vi "Derivative (single).vi"(8 "error in (no error)":errorcluster, 9 "Type":enum16{"dy/dx vs x", "dx/dy vs y"}(ring), 11 "XY-data":cluster{"X-array":dbl[], "Y-array":dbl[]}) -> (0 "error out":errorcluster, 2 "Differential out":cluster{"X-array":dbl[], "Y-array":dbl[]} {"Y-array" format="%.2p"; "X-array" format="%.2p"}, 3 "XY-data out":cluster{"X-array":dbl[], "Y-array":dbl[]})   [LabVIEW 2019, in "xy_utilities.lvlib"]
doc: "Performs numerical differentiation of <b>XY-data</b> using the finite difference method.\n\n<b>Interval</b> is the range over which the finite difference is calculated.\n<b>Interval Units</b> defines the units of the <b>Interval</b> to be the number of points or the same units as the x (or y) data.\n<b>Type</b> specifies taking a derivative with respect to x or y.\n\nWire data to the data input to determine the polymorphic instance to use or manually select the instance."
uses:
  xy_utilities.lvlib
  <vilib>/Analysis/NI_AALPro.lvlib
  Swap X and Y (single).vi
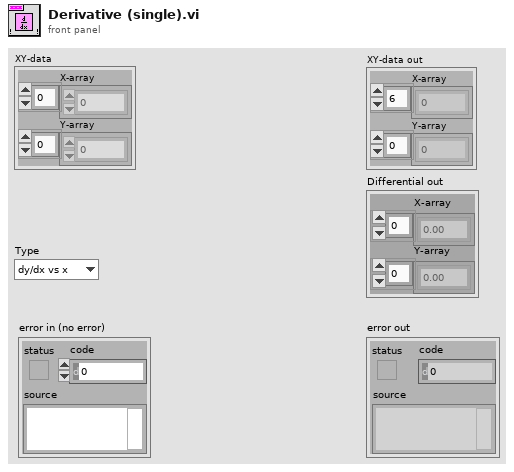
[diagram p1: front panel]
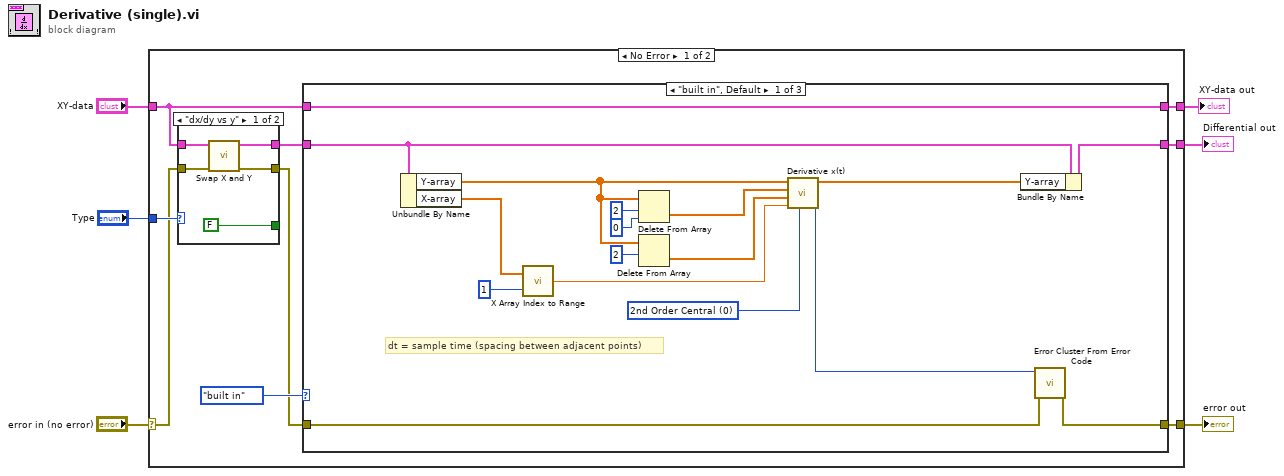
[diagram p0: block diagram]
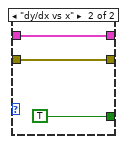
[diagram p2: hidden frame]
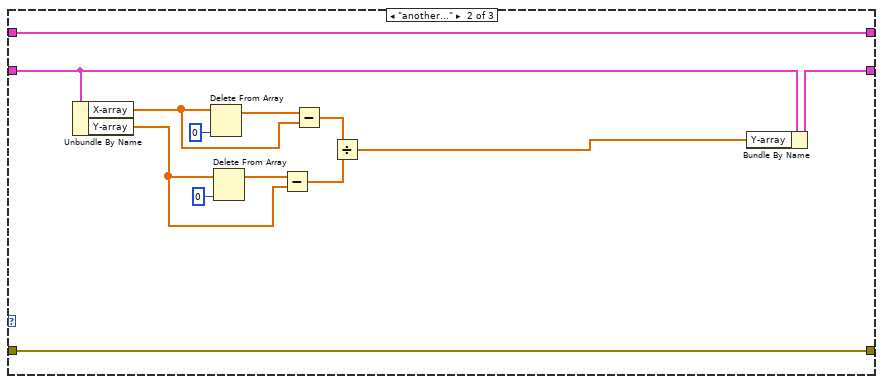
[diagram p3: hidden frame]
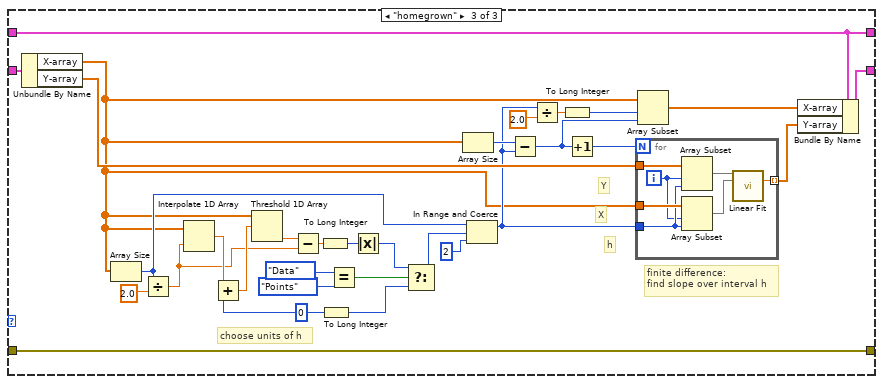
[diagram p4: hidden frame]
diagram:
  n1 = case shown="No Error" "error in (no error)" {
    selector: "error in (no error)" -> [w14 w93]
    tunnel: [w9 w93] -> w5
    tunnel: "XY-data" -> [w13 w92]
    tunnel: [w12 _] -> w3
    tunnel: "Type" -> [w15 _]
    tunnel: [w10 w92] -> w1
    frame No Error {
      n2 = case shown="\"dx/dy vs y\"" w15 {
        tunnel: w13 -> [w20 w23]
        tunnel: [w19 w23] -> w11
        tunnel: [w18 w22] -> w7
        tunnel: w14 -> [w17 w22]
        tunnel: [FALSE ("dy/dx vs x") TRUE ("dy/dx vs x")] -> _
        frame "dx/dy vs y" {
          n3 = call-poly "Swap X and Y.vi"("error in (no error)"=w17, "XY-data"=w20) -> ("error out"=w18:errorcluster, "XY-data out"=w19:cluster{"X-array":dbl[], "Y-array":dbl[]})  [unwired: 8 in]
        }
        frame "dy/dx vs x" {
        }
      }
      n4 = case shown="\"built in\", Default" enum16{"built in", "another...", "homegrown"}."built in" ("Subset Method") {
        tunnel: w13 -> [w37 w52 w67]
        tunnel: [w36 w44 w54] -> w12
        tunnel: w11 -> [w38 w46 w55]
        tunnel: [w37 w52 w67] -> w10
        tunnel: [w39 w53 w66] -> w9
        tunnel: w7 -> [w40 w53 w66]
        frame "built in", Default {
          w31 = u16 0 items=["2nd Order Central", "4th Order Central", "Forward", "Backward"] ("method")
          # "dt = sample time (spacing between adjacent points)"
          n5 = Unbundle By Name(w38) -> ("Y-array"=w30:dbl[], "X-array"=w35:dbl[])
          n6 = call "X Array Index to Range.vi"("X Range (points)"=1 ("X Range (index)"), "X-array"=w35) -> ("X Range (data)"=w34:dbl)
          n7 = Delete From Array(array=w30, length=2 ("index"), index=0 ("length")) -> (deleted portion=w33:dbl[])  [unwired: 1 out]
          n8 = Delete From Array(array=w30, length=2 ("index")) -> (deleted portion=w26:dbl[])  [unwired: 1 in, 1 out]
          n9 = call <vilib>:"Derivative x(t).vi"("method"=w31, "dt"=w34, "Final Condition"=w26, "Initial Condition"=w33, "X"=w30) -> ("error"=w32:i32, "dX/dt"=w25:dbl[])  [unwired: 5 in]
          n10 = Bundle By Name(cluster=w38, "Y-array"=w25) -> (w36:cluster{"X-array":dbl[], "Y-array":dbl[]})
          n11 = call <vilib>:"Error Cluster From Error Code.vi"("error in (no error)"=w40, "error code (0)"=w32) -> ("error out"=w39:errorcluster)  [unwired: 7 in]
        }
        frame "another..." {
          n12 = Unbundle By Name(w46) -> ("X-array"=w41:dbl[], "Y-array"=w49:dbl[])
          n13 = Delete From Array(array=w41, index=0) -> (array with subset deleted=w51:dbl[])  [unwired: 1 in, 1 out]
          n14 = Delete From Array(array=w49, index=0) -> (array with subset deleted=w50:dbl[])  [unwired: 1 in, 1 out]
          n15 = Subtract(x=w50, y=w49) -> (x-y=w47:dbl[])
          n16 = Subtract(x=w51, y=w41) -> (x-y=w48:dbl[])
          n17 = Divide(x=w48, y=w47) -> (x/y=w45:dbl[])
          n18 = Bundle By Name(cluster=w46, "Y-array"=w45) -> (w44:cluster{"X-array":dbl[], "Y-array":dbl[]})
        }
        frame "homegrown" {
          w56 = 0 ("number")
          # "choose units of h"
          # "h"
          # "finite difference:\nfind slope over interval h"
          # "Y"
          # "X"
          n19 = Unbundle By Name(w55) -> ("X-array"=w58:dbl[], "Y-array"=w68:dbl[])
          n20 = Array Size(array=w58) -> (size(s)=w65:i32)
          n21 = Divide(x=w65, y=2.0) -> (x/y=w59:dbl)
          n22 = Interpolate 1D Array(1:w59, 2:w58) -> (0:w60:dbl)
          n23 = Add(x=w60, y=w56) -> (x+y=w74:dbl)
          n24 = Threshold 1D Array(2:w74, 3:w58) -> (0:w76:dbl)  [unwired: 1 in]
          n25 = Subtract(x=w76, y=w59) -> (x-y=w75:dbl)
          n26 = To Long Integer(number=w75) -> (32bit integer=w73:i32)
          n27 = To Long Integer(number=w56) -> (32bit integer=w70:i32)
          n28 = Equal?(x=enum16{"Points", "Data"}."Data" ("Interval Units"), y=enum16{"Points", "Data"}."Points") -> (x = y?=w71:bool)
          n29 = Absolute Value(x=w73) -> (abs(x)=w63:i32)
          n30 = Select(t=w63, s=w71, f=w70) -> (s? t:f=w62:i32)
          n31 = Array Size(array=w58) -> (size(s)=w80:i32)
          n32 = In Range and Coerce(upper limit=w65, x=w62, lower limit=2) -> (coerced(x)=w61:i32)  [unwired: 1 out]
          n33 = Subtract(x=w80, y=w61) -> (x-y=w83:i32)
          n34 = Divide(x=w61, y=2.0) -> (x/y=w78:dbl)
          n35 = To Long Integer(number=w78) -> (32bit integer=w84:i32)
          n36 = Increment(x=w83) -> (x+1=w81:i32)
          n37 = for {
            N: w81 -> [_]
            tunnel: w68 -> [w91]
            tunnel: w58 -> [w90]
            tunnel: w61 -> [w89]
            tunnel: [w88] -> w69 mode=indexing
            i -> [w85]
            n38 = Array Subset "Array Subset"(array=w91, index=w85, length=w89) -> (w87:dbl[])
            n39 = Array Subset(array=w90, index=w85, length=w89) -> (w86:dbl[])
            n40 = call <vilib>:"Linear Fit.vi"("Y"=w87, "X"=w86) -> ("slope"=w88:dbl)  [unwired: 9 in, 4 out]
          }
          n41 = Array Subset(array=w58, index=w84, length=w83) -> (w82:dbl[])
          n42 = Bundle By Name(cluster=w67, "X-array"=w82, "Y-array"=w69) -> (w54:cluster{"X-array":dbl[], "Y-array":dbl[]})
        }
      }
    }
    frame Error {
    }
  }
  "error out" <- w5
  "Differential out" <- w3
  "XY-data out" <- w1
